vi "SpeedController_Final2.0.vi"() -> ()   [LabVIEW 2020]
panel:
  out "Safety Govenor Active":bool
  out "Access Granted 2":bool
  out "Intruder Alert 2":bool
  out "Voice Command":string
  out "String":string
  in  "Module Path":path
  in  "Stop 2":bool
  out "BREAKING":bool
  out "ERROR OUT":errorcluster
  out "SPEED OVERRIDE WARNING":bool
  out "Safety Speed Cap":dbl
  out "Live Light Level (ADC)":dbl
  in  "Requested Speed (Delay)":dbl(slide) scale=800.0..3000.0
  in  "Stop 1":bool
  in  "VISA Resource Name":refnum<visa-resource-name>
  # "OUTPUTS & INDICATORS"
  # "Voice Access"
  # "INPUTS"
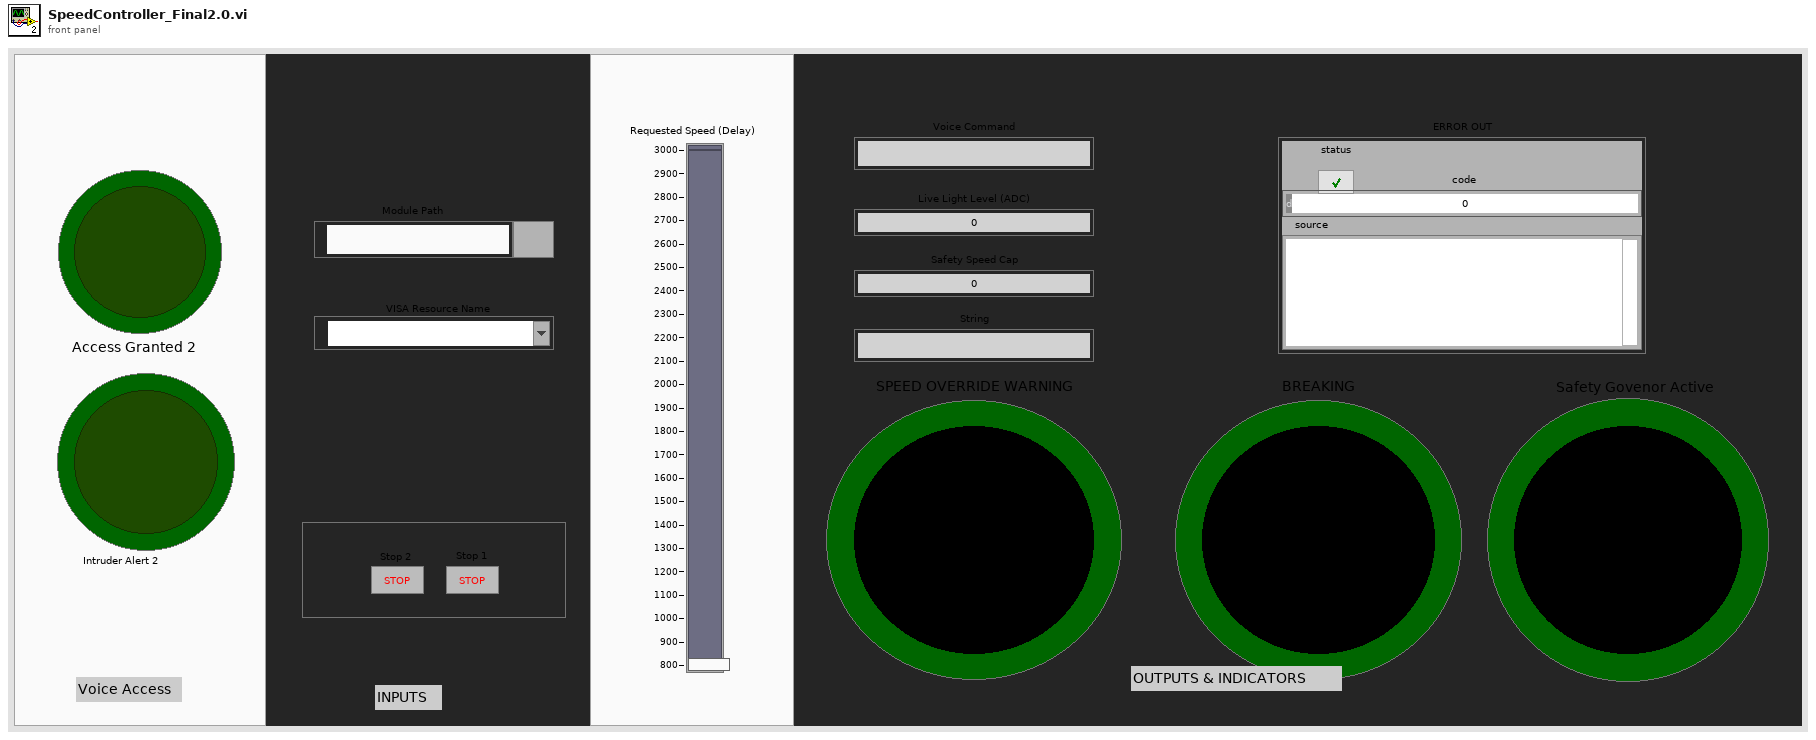
[diagram p1: front panel]
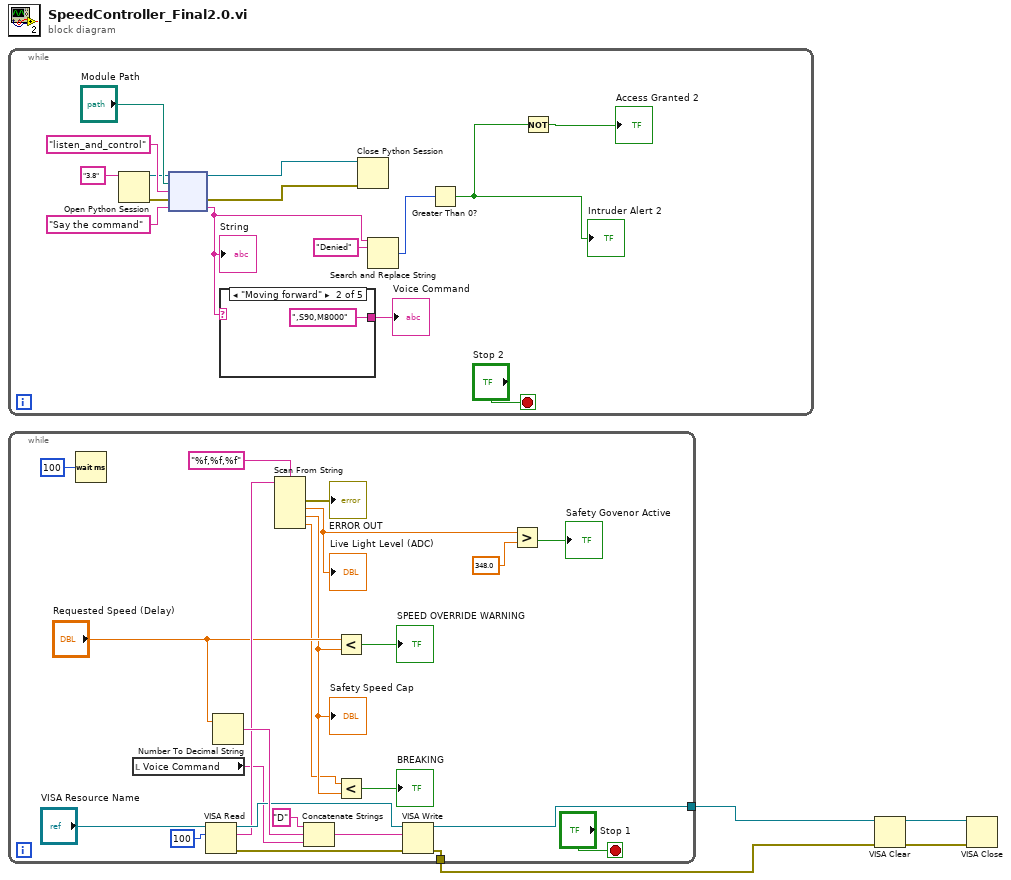
[diagram p0: block diagram]
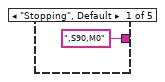
[diagram p2: hidden frame]
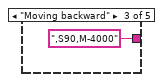
[diagram p3: hidden frame]
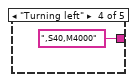
[diagram p4: hidden frame]
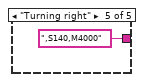
[diagram p5: hidden frame]
diagram:
  n1 = while {
    stop <- "Stop 2" stop-if-true
    n2 = Open Python Session(python version="3.8" ("Python version")) -> (session out=w15:refnum<k35>, error out=w14:errorcluster)  [unwired: 2 in]
    n3 = node(w15, "Module Path", "listen_and_control" ("function name"), w14, "Say the command") -> (w16:refnum<k35>, w13:errorcluster, w5:string)  [unwired: 2 out]
    "String" <- w5
    n4 = case shown="\"Moving forward\"" w5 {
      tunnel: [",S90,M0" ",S90,M8000" ",S90,M-4000" ",S40,M4000" ",S140,M4000"] -> w10
      frame "Stopping", Default {
      }
      frame "Moving forward" {
      }
      frame "Moving backward" {
      }
      frame "Turning left" {
      }
      frame "Turning right" {
      }
    }
    "Voice Command" <- w10
    n5 = Close Python Session(session in=w16, error in=w13) -> ()  [unwired: 1 out]
    n6 = Search and Replace String(input string=w5, search string="Denied") -> (number of replacements=w8:i32)  [unwired: 6 in, 3 out]
    n7 = Greater Than 0?(x=w8) -> (x > 0?=w6:bool)
    "Intruder Alert 2" <- w6
    n8 = Not(x=w6) -> (.not. x?=→"Access Granted 2":bool)
  }
  n9 = while {
    tunnel: [w31] -> w4
    tunnel: [w30] -> w3
    stop <- "Stop 1" stop-if-true
    n10 = Wait (ms)(milliseconds to wait=u32 100) -> ()  [unwired: 1 out]
    n11 = local read "Voice Command"() -> (w32:string)
    n12 = VISA Read(VISA resource name="VISA Resource Name", byte count=u32 100) -> (VISA resource name out=w44:refnum<visa-resource-name>, read buffer=w38:string, error out=w43:errorcluster)  [unwired: 1 in, 1 out]
    n13 = Number To Decimal String(number="Requested Speed (Delay)") -> (decimal integer string=w46:string)  [unwired: 1 in]
    n14 = Scan From String(format string="%f,%f,%f", input string=w38) -> (error out=→"ERROR OUT":errorcluster, output 1=w27:dbl, output 2=w29:dbl, output 3=w28:dbl)  [unwired: 5 in, 2 out]
    "Live Light Level (ADC)" <- w27
    "Safety Speed Cap" <- w29
    n15 = Concatenate Strings("D" ("string"), w46, w32) -> (w45:string)
    n16 = Less?(x="Requested Speed (Delay)", y=w29) -> (x < y?=→"SPEED OVERRIDE WARNING":bool)
    n17 = Less?(x=w28, y=w29) -> (x < y?=→"BREAKING":bool)
    n18 = VISA Write(VISA resource name=w44, write buffer=w45, error in (no error)=w43) -> (VISA resource name out=w30:refnum<visa-resource-name>, error out=w31:errorcluster)  [unwired: 1 out]
    n19 = Greater?(x=w27, y=348.0) -> (0:→"Safety Govenor Active":bool)
  }
  n20 = VISA Clear(VISA resource name=w3, error in (no error)=w4) -> (VISA resource name out=w2:refnum<visa-resource-name>, error out=w1:errorcluster)
  n21 = VISA Close(VISA resource name=w2, error in (no error)=w1) -> ()  [unwired: 1 out]
